vi "PatterningProgramV2.vi"() -> ()   [LabVIEW 2023]
uses:
  <vilib>/Platform/TimedLoop/XDataNode/timing_clust.ctl
  <vilib>/Platform/TimedLoop/XDataNode/nitl_modes.ctl
  <vilib>/Platform/TimedLoop/XDataNode/wakeup.ctl
  <vilib>/DAQmx/write.llb/DAQmx Write (Digital Bool 1Line 1Point).vi
  <vilib>/DAQmx/create/channels.llb/DAQmx Create Channel (DO-Digital Output).vi
  <vilib>/DAQmx/miscellaneous.llb/DAQmx Fill In Error Info.vi
  <vilib>/Platform/TimedLoop/XDataNode/XDataNode.xnode
  <vilib>/Platform/TimedLoop/XDataNode/XDNodeRunTimeDep.lvlib
  C:/Program Files (x86)/Control/SC3U.dll
  Program Files (x86)/Control/SC3U.dll
panel:
  out "Patterns Left":dbl
  out "Z Focus Positions":dbl[](array[numeric])
  out "Y Focus Positions":dbl[](array[numeric])
  out "X Focus Positions":dbl[](array[numeric])
  in  "Focus Position 4":bool
  in  "Focus Position 3":bool
  in  "Focus Position 2":bool
  in  "Focus Position 1":bool
  in  "stop":bool
  in  "450 nm":bool
  out "Boolean 3":bool
  in  "617 nm":bool
  out "Boolean 4":bool
  out "Patterning Time":dbl
  out "Pattern Spacing (mm)":dbl
  out "Well Spacing":dbl caption="Well Spacing (mm)"
  in  "START":bool
  in  "Pattern Time (s)":dbl=0.5 min=0.1 max=900.0
  in  "Well Columns":dbl=1.0 min=1.0 step=1.0
  in  "Well Rows":dbl=1.0 min=1.0 step=1.0
  in  "Pattern Columns":dbl=1.0 min=1.0 max=100.0 step=1.0
  in  "Pattern Rows":dbl=1.0 min=1.0 max=100.0 step=1.0
  in  "Select Objective Lens":u16(ring) items=["4X", "10X", "20X", "40X"]
  in  "Select Well Vessel":u16(ring) items=["Single Well", "6-Well Plate", "12-Well Plate", "24-Well Plate", "96-Well Plate"]
  in  "SC3U":refnum<k24>(container)
  out "ConnectStatus":bool
  out "ComUsing":i16
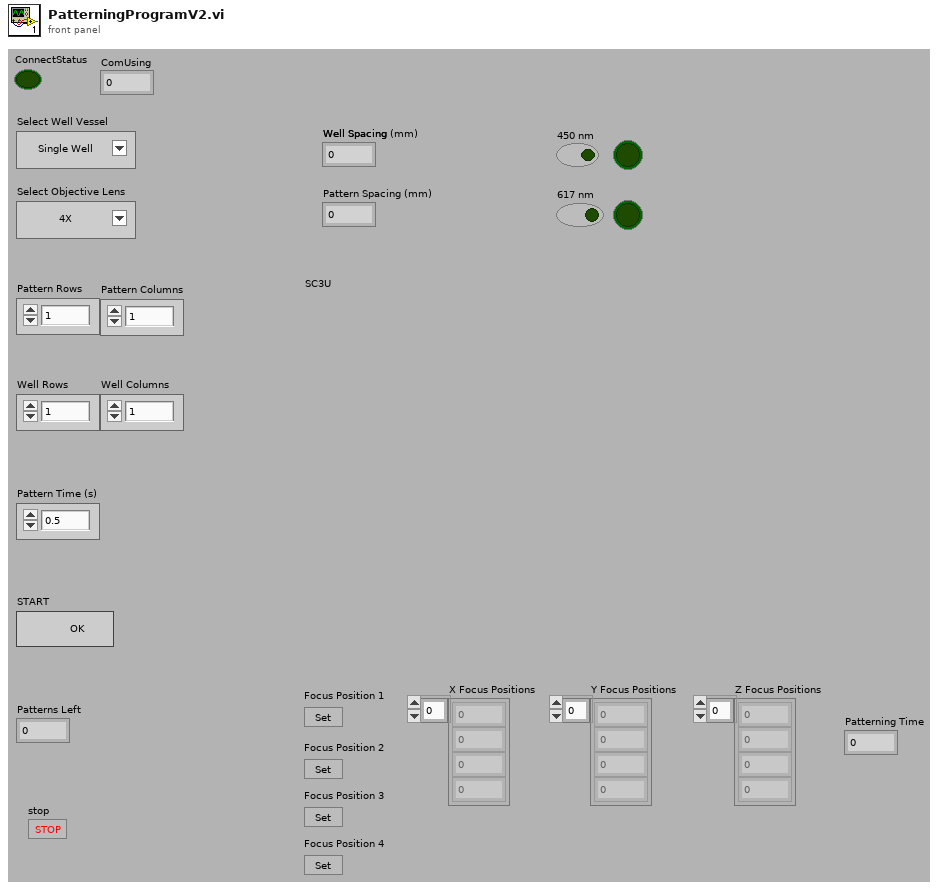
[diagram p1: front panel]
types:
  T1 = typedef "XDNodeRunTimeDep.lvlib/timing_clust.ctl" = cluster{"Expected End [f-1]":u64, "Actual End [f-1]":u64, "Finished Late? [f-1]":bool, "Expected End [i-1]":u64, "Actual End [i-1]":u64, "Finished Late? [i-1]":bool, "Expected Start [i]":u64, "Actual Start [i]":u64, "Expected Start [f]":u64, "Actual Start [f]":u64, "Source Name":string, "Structure Name":string, "Period":i64, "Deadline":i64, "Offset":i64, "Start":i64, "Priority":i32, "Timeout":i32, "Mode":T2, "Wakeup Reason":T3, "Error":errorcluster, "Source Type":string, "Secondary Source Type":string, "Global End Time":u64, "Global Start Time":u64, "Frame Duration":u64, "Iteration Duration":u64, "Assigned CPU":i32, "I/O Scan Engine Mode":u32}
  T2 = typedef "XDNodeRunTimeDep.lvlib/nitl_modes.ctl" = enum32{"No Change", "Process missed periods, maintain original phase", "Discard missed periods, maintain original phase", "Process missed periods, ignore original phase", "Discard missed periods, ignore original phase"}
  T3 = typedef "XDNodeRunTimeDep.lvlib/wakeup.ctl" = enum32{"Normal", "Aborted", "Asynchronous wakeup", "Timing source error", "Timed loop error", "Timeout"}
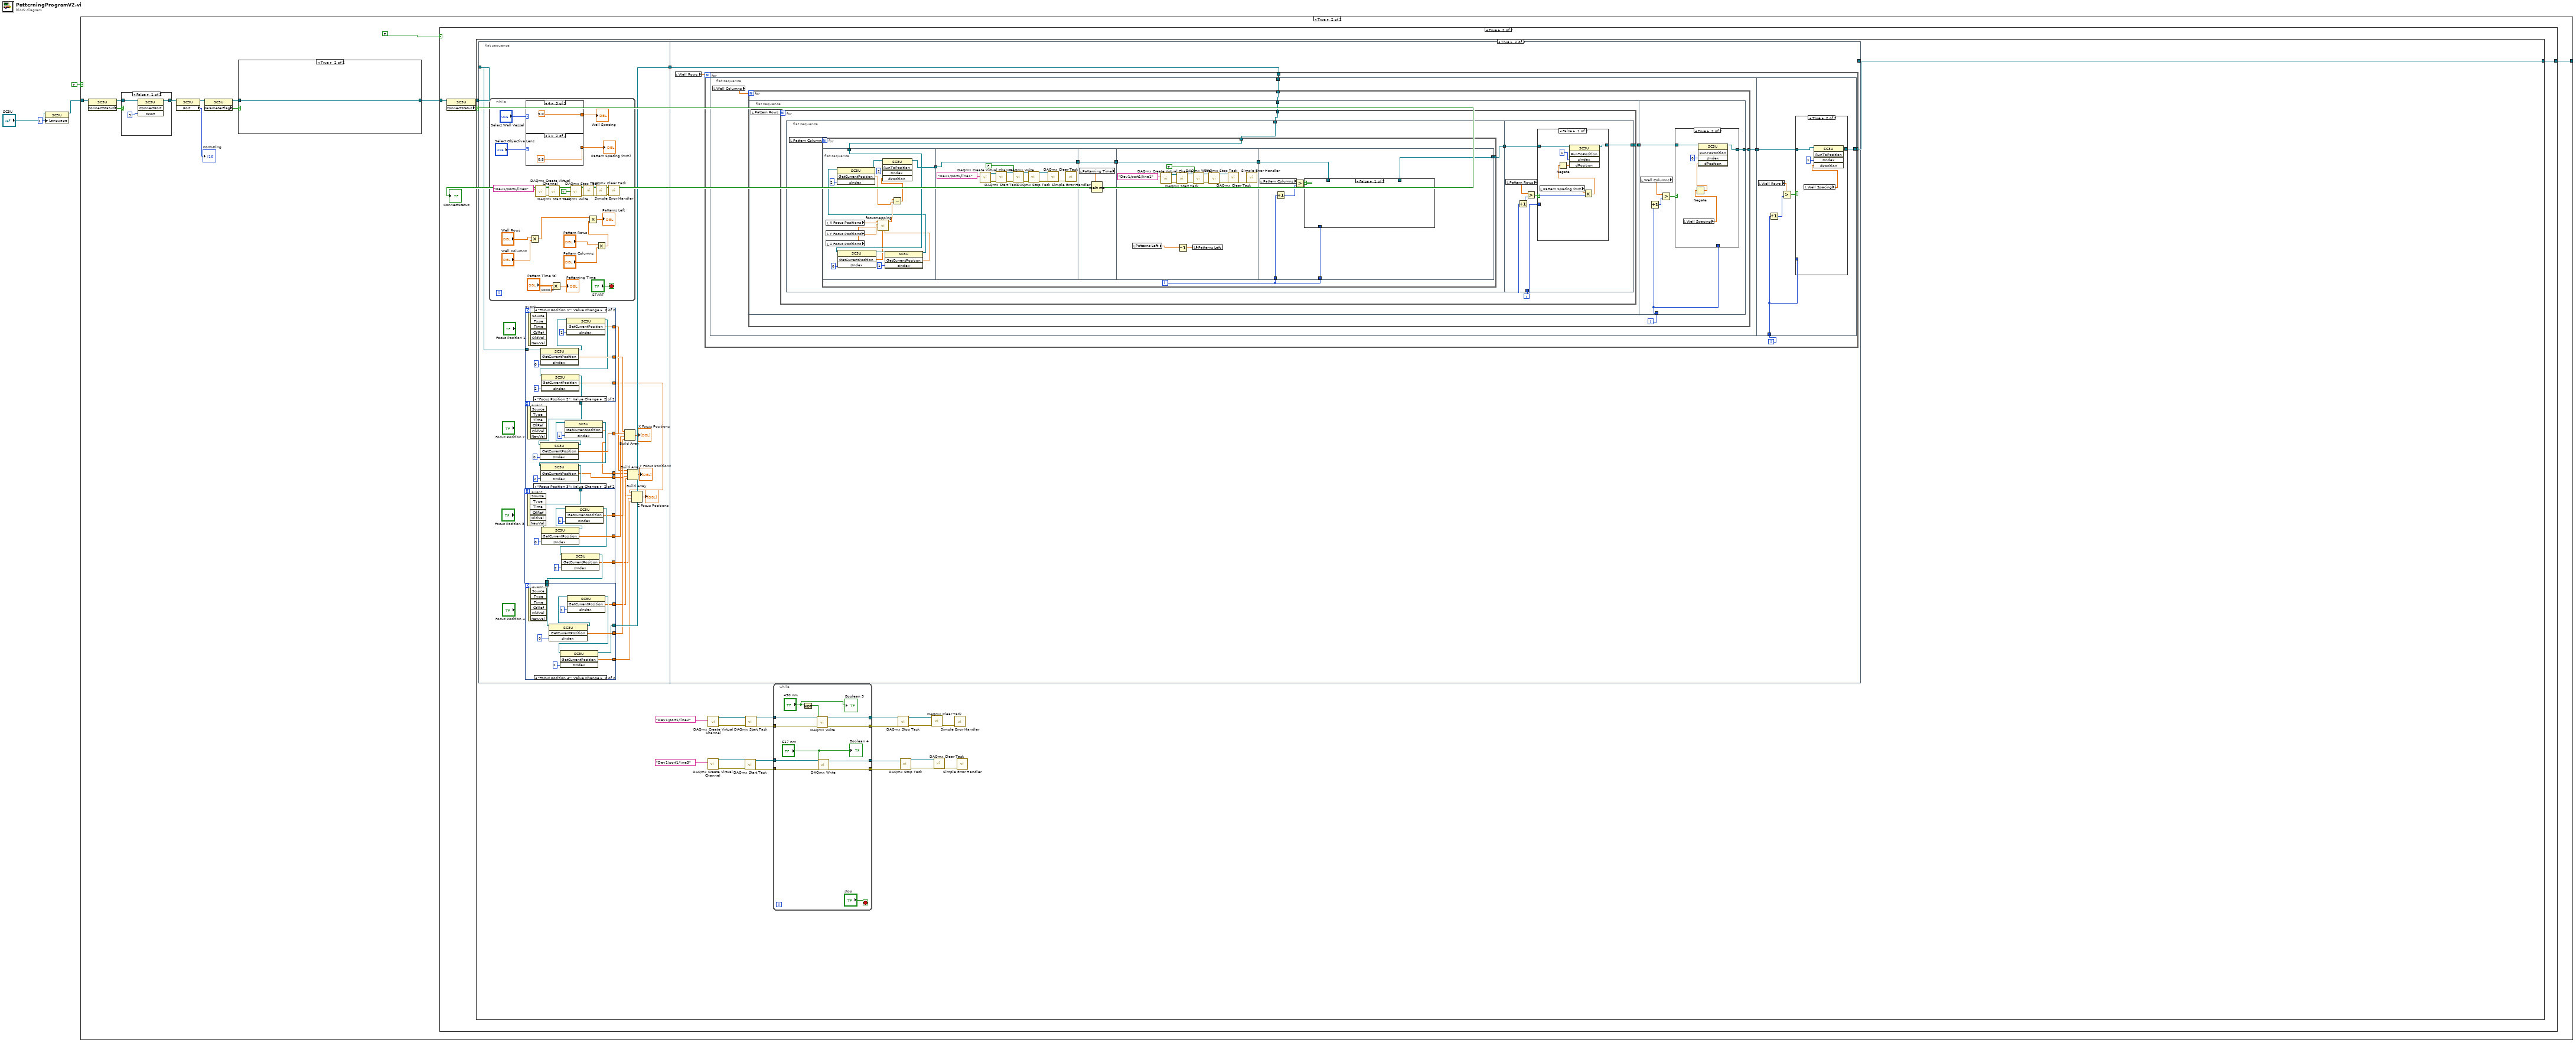
[diagram p0: block diagram]
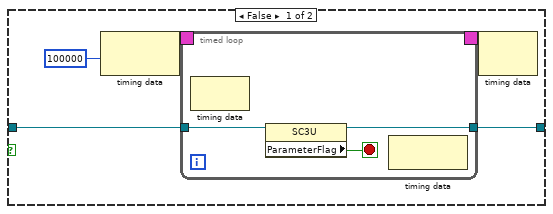
[diagram p3: hidden frame]
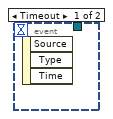
[diagram p7: hidden frame]
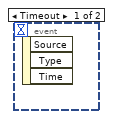
[diagram p8: hidden frame]
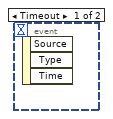
[diagram p9: hidden frame]
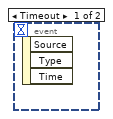
[diagram p10: hidden frame]
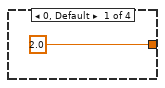
[diagram p11: hidden frame]
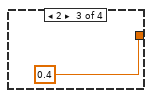
[diagram p12: hidden frame]
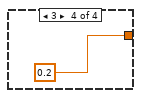
[diagram p13: hidden frame]
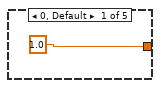
[diagram p14: hidden frame]
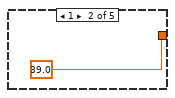
[diagram p15: hidden frame]
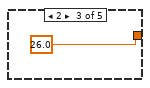
[diagram p16: hidden frame]
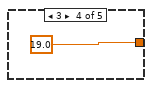
[diagram p17: hidden frame]
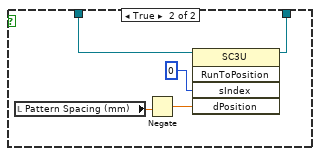
[diagram p18: hidden frame]
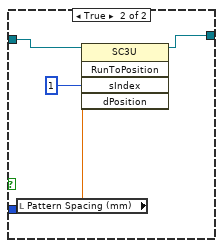
[diagram p19: hidden frame]
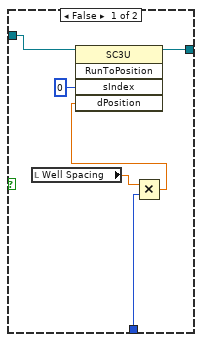
[diagram p20: hidden frame]
diagram:
  n1 = property class="SC3U"(reference="SC3U", "Language"=i16 1 ("intLanguage")) -> (reference out=w2:refnum<k24>)  [unwired: 1 in, 1 out]
  n2 = case shown="True" TRUE {
    tunnel: [_ w15] -> _
    tunnel: w2 -> [_ w13]
    frame False {
    }
    frame True {
      n3 = property class="SC3U"(reference=w13) -> (reference out=w12:refnum<k24>, "ConnectStatus"=w11:bool)  [unwired: 1 in, 1 out]
      n4 = case shown="False" w11 {
        tunnel: w12 -> [w33 w34]
        tunnel: [w32 w34] -> w10
        frame False {
          n5 = invoke class="SC3U" method="ConnectPort"(reference=w33, "sPort"=i16 5 ("ComUsing")) -> (reference out=w32:refnum<k24>)  [unwired: 2 in, 3 out]
        }
        frame True {
        }
      }
      n6 = property class="SC3U"(reference=w10) -> (reference out=w8:refnum<k24>, "Port"=→"ComUsing":i16)  [unwired: 1 in, 1 out]
      n7 = property class="SC3U"(reference=w8) -> (reference out=w7:refnum<k24>, "ParameterFlag"=w6:bool)  [unwired: 1 in, 1 out]
      n8 = case shown="True" w6 {
        tunnel: w7 -> [w17 w30]
        tunnel: [w16 w30] -> w14
        frame False {
          n9 = node-c288(i64 100000 ("周期")) -> (w20:T1)
          n10 = timed-loop {
            timing: w20 -> [_]
            timing-out: [_] -> w19
            tunnel: w17 -> [w23]
            tunnel: [w22] -> w16
            stop <- w21 stop-if-true
            n11 = node-c288() -> ()  [unwired: 1 in, 1 out]
            n12 = property class="SC3U"(reference=w23) -> (reference out=w22:refnum<k24>, "ParameterFlag"=w21:bool)  [unwired: 1 in, 1 out]
            n13 = node-c288() -> ()  [unwired: 1 in, 1 out]
          }
          n14 = node-c288(w19) -> ()  [unwired: 1 out]
        }
        frame True {
        }
      }
      n15 = case shown="True" TRUE {
        tunnel: w14 -> [_ w37]
        tunnel: [_ w38] -> w15
        frame False {
        }
        frame True {
          n16 = property class="SC3U"(reference=w37) -> (reference out=w36:refnum<k24>, "ConnectStatus"=w35:bool)  [unwired: 1 in, 1 out]
          "ConnectStatus" <- w35
          n17 = case shown="True" w35 {
            tunnel: w36 -> [_ w61]
            tunnel: [_ w59] -> w38
            frame False {
            }
            frame True {
              n18 = flat-sequence {
                tunnel: w61 -> [w93]
                tunnel: [w87] -> w60
                tunnel: w60 -> [w170]
                tunnel: [w169] -> w59
                frame #0 {
                  n19 = while {
                    stop <- "START" stop-if-true
                    n20 = case shown="1" "Select Objective Lens" {
                      tunnel: [2.0 ("Numeric") 0.8 ("Numeric") 0.4 ("Numeric") 0.2 ("Numeric")] -> w155
                      frame 0, Default {
                      }
                      frame 1 {
                      }
                      frame 2 {
                      }
                      frame 3 {
                      }
                    }
                    "Pattern Spacing (mm)" <- w155
                    n21 = case shown="4" "Select Well Vessel" {
                      tunnel: [1.0 ("Numeric") 39.0 ("Numeric") 26.0 ("Numeric") 19.0 ("Numeric") 9.0 ("Numeric")] -> w157
                      frame 0, Default {
                      }
                      frame 1 {
                      }
                      frame 2 {
                      }
                      frame 3 {
                      }
                      frame 4 {
                      }
                    }
                    "Well Spacing" <- w157
                    n22 = Multiply(x="Well Rows", y="Well Columns") -> (x*y=w136:dbl)
                    n23 = call-poly <vilib>:"DAQmx Create Virtual Channel.vi"("lines"=tag "Dev1/port1/line0") -> ("task out"=w151:refnum<k21>, "error out"=w149:errorcluster)  [unwired: 13 in]
                    n24 = call <vilib>:"DAQmx Start Task.vi"("task/channels in"=w151, "error in"=w149) -> ("task out"=w146:refnum<k21>, "error out"=w145:errorcluster)  [unwired: 12 in]
                    n25 = Multiply(x="Pattern Time (s)", y=1000.0) -> (x*y=→"Patterning Time":dbl)
                    n26 = call-poly <vilib>:"DAQmx Write.vi"("task/channels in"=w146, "data"=TRUE, "error in"=w145) -> ("task out"=w144:refnum<k21>, "error out"=w143:errorcluster)  [unwired: 10 in, 1 out]
                    n27 = call <vilib>:"DAQmx Stop Task.vi"("task/channels in"=w144, "error in"=w143) -> ("task out"=w150:refnum<k21>, "error out"=w148:errorcluster)  [unwired: 12 in]
                    n28 = call <vilib>:"DAQmx Clear Task.vi"("task in"=w150, "error in"=w148) -> ("error out"=w147:errorcluster)  [unwired: 13 in]
                    n29 = Multiply(x="Pattern Rows", y="Pattern Columns") -> (x*y=w135:dbl)
                    n30 = Multiply(x=w136, y=w135) -> (x*y=→"Patterns Left":dbl)
                    n31 = call <vilib>:"Simple Error Handler.vi"("error in (no error)"=w147) -> ()  [unwired: 4 in, 5 out]
                  }
                  n32 = event shown="[1] \"Focus Position 1\": Value Change" {
                    selector: _ -> [_ _]
                    dyn-events: _ -> [_ _]
                    timeout: _ -> [_ _]
                    tunnel: w93 -> [_ w132]
                    tunnel: [_ w131] -> w92
                    tunnel: [_ w126] -> w91
                    tunnel: [_ w125] -> w83
                    tunnel: [_ w124] -> w78
                    event Timeout {
                      n33 = event-data() -> ()  [unwired: 1 in, 3 out]
                    }
                    event "Focus Position 1": Value Change {
                      n34 = event-data() -> ()  [unwired: 1 in, 6 out]
                      n35 = invoke class="SC3U" method="GetCurrentPosition"(reference=w132, "sIndex"=i16 0) -> (reference out=w128:refnum<k24>, "GetCurrentPosition"=w131:dbl)  [unwired: 2 in, 2 out]
                      n36 = invoke class="SC3U" method="GetCurrentPosition"(reference=w128, "sIndex"=i16 1) -> (reference out=w127:refnum<k24>, "GetCurrentPosition"=w125:dbl)  [unwired: 2 in, 2 out]
                      n37 = invoke class="SC3U" method="GetCurrentPosition"(reference=w127, "sIndex"=i16 2) -> (reference out=w126:refnum<k24>, "GetCurrentPosition"=w124:dbl)  [unwired: 2 in, 2 out]
                    }
                  }
                  n38 = event shown="[1] \"Focus Position 2\": Value Change" {
                    selector: _ -> [_ _]
                    dyn-events: _ -> [_ _]
                    timeout: _ -> [_ _]
                    tunnel: w91 -> [_ w122]
                    tunnel: [_ w121] -> w90
                    tunnel: [_ w116] -> w89
                    tunnel: [_ w115] -> w82
                    tunnel: [_ w114] -> w77
                    event Timeout {
                      n39 = event-data() -> ()  [unwired: 1 in, 3 out]
                    }
                    event "Focus Position 2": Value Change {
                      n40 = event-data() -> ()  [unwired: 1 in, 6 out]
                      n41 = invoke class="SC3U" method="GetCurrentPosition"(reference=w122, "sIndex"=i16 0) -> (reference out=w118:refnum<k24>, "GetCurrentPosition"=w121:dbl)  [unwired: 2 in, 2 out]
                      n42 = invoke class="SC3U" method="GetCurrentPosition"(reference=w118, "sIndex"=i16 1) -> (reference out=w117:refnum<k24>, "GetCurrentPosition"=w115:dbl)  [unwired: 2 in, 2 out]
                      n43 = invoke class="SC3U" method="GetCurrentPosition"(reference=w117, "sIndex"=i16 2) -> (reference out=w116:refnum<k24>, "GetCurrentPosition"=w114:dbl)  [unwired: 2 in, 2 out]
                    }
                  }
                  n44 = event shown="[1] \"Focus Position 3\": Value Change" {
                    selector: _ -> [_ _]
                    dyn-events: _ -> [_ _]
                    timeout: _ -> [_ _]
                    tunnel: w89 -> [_ w112]
                    tunnel: [_ w106] -> w88
                    tunnel: [_ w111] -> w86
                    tunnel: [_ w105] -> w81
                    tunnel: [_ w104] -> w76
                    event Timeout {
                      n45 = event-data() -> ()  [unwired: 1 in, 3 out]
                    }
                    event "Focus Position 3": Value Change {
                      n46 = event-data() -> ()  [unwired: 1 in, 6 out]
                      n47 = invoke class="SC3U" method="GetCurrentPosition"(reference=w112, "sIndex"=i16 0) -> (reference out=w108:refnum<k24>, "GetCurrentPosition"=w111:dbl)  [unwired: 2 in, 2 out]
                      n48 = invoke class="SC3U" method="GetCurrentPosition"(reference=w108, "sIndex"=i16 1) -> (reference out=w107:refnum<k24>, "GetCurrentPosition"=w105:dbl)  [unwired: 2 in, 2 out]
                      n49 = invoke class="SC3U" method="GetCurrentPosition"(reference=w107, "sIndex"=i16 2) -> (reference out=w106:refnum<k24>, "GetCurrentPosition"=w104:dbl)  [unwired: 2 in, 2 out]
                    }
                  }
                  n50 = event shown="[1] \"Focus Position 4\": Value Change" {
                    selector: _ -> [_ _]
                    dyn-events: _ -> [_ _]
                    timeout: _ -> [_ _]
                    tunnel: w88 -> [_ w102]
                    tunnel: [_ w96] -> w87
                    tunnel: [_ w101] -> w85
                    tunnel: [_ w95] -> w80
                    tunnel: [_ w94] -> w75
                    event Timeout {
                      n51 = event-data() -> ()  [unwired: 1 in, 3 out]
                    }
                    event "Focus Position 4": Value Change {
                      n52 = event-data() -> ()  [unwired: 1 in, 6 out]
                      n53 = invoke class="SC3U" method="GetCurrentPosition"(reference=w102, "sIndex"=i16 0) -> (reference out=w98:refnum<k24>, "GetCurrentPosition"=w101:dbl)  [unwired: 2 in, 2 out]
                      n54 = invoke class="SC3U" method="GetCurrentPosition"(reference=w98, "sIndex"=i16 1) -> (reference out=w97:refnum<k24>, "GetCurrentPosition"=w95:dbl)  [unwired: 2 in, 2 out]
                      n55 = invoke class="SC3U" method="GetCurrentPosition"(reference=w97, "sIndex"=i16 2) -> (reference out=w96:refnum<k24>, "GetCurrentPosition"=w94:dbl)  [unwired: 2 in, 2 out]
                    }
                  }
                  n56 = Build Array(w92, w90, w86, w85) -> (→"X Focus Positions":dbl[])
                  n57 = Build Array(w83, w82, w81, w80) -> (→"Y Focus Positions":dbl[])
                  n58 = Build Array(w78, w77, w76, w75) -> (→"Z Focus Positions":dbl[])
                }
                frame #1 {
                  n59 = local read "Well Rows"() -> (w171:dbl)
                  n60 = for {
                    N: w171 -> [_]
                    tunnel: [w173] -> w169
                    tunnel: w170 -> [w172]
                    i -> [w175]
                    n61 = flat-sequence {
                      tunnel: [w177] -> w174
                      tunnel: w172 -> [w176]
                      tunnel: w175 -> [w299]
                      tunnel: w174 -> [w298]
                      tunnel: [w297] -> w173
                      frame #0 {
                        n62 = local read "Well Columns"() -> (w178:dbl)
                        n63 = for {
                          N: w178 -> [_]
                          tunnel: w176 -> [w182]
                          tunnel: [w179] -> w177
                          i -> [w181]
                          n64 = flat-sequence {
                            tunnel: w182 -> [w184]
                            tunnel: [w183] -> w180
                            tunnel: w181 -> [w281]
                            tunnel: w180 -> [w282]
                            tunnel: [w280] -> w179
                            frame #0 {
                              n65 = local read "Pattern Rows"() -> (w185:dbl)
                              n66 = for {
                                N: w185 -> [_]
                                tunnel: w184 -> [w189]
                                tunnel: [w186] -> w183
                                i -> [w188]
                                n67 = flat-sequence {
                                tunnel: w189 -> [w191]
                                tunnel: [w190] -> w187
                                tunnel: w188 -> [w265]
                                tunnel: w187 -> [w264]
                                tunnel: [w263] -> w186
                                frame #0 {
                                n68 = local read "Pattern Columns"() -> (w192:dbl)
                                n69 = for {
                                N: w192 -> [_]
                                tunnel: w191 -> [w197]
                                tunnel: [w199] -> w190
                                i -> [w198]
                                n70 = flat-sequence {
                                tunnel: w197 -> [w204]
                                tunnel: [w215] -> w193
                                tunnel: [w217] -> w194
                                tunnel: w193 -> [w217]
                                tunnel: [w229] -> w195
                                tunnel: w194 -> [w229]
                                tunnel: [w233] -> w196
                                tunnel: w195 -> [w233]
                                tunnel: w198 -> [w247]
                                tunnel: [w249] -> w199
                                tunnel: w198 -> [w248]
                                tunnel: w196 -> [w245]
                                frame #0 {
                                n71 = local read "X Focus Positions"() -> (w210:dbl[])
                                n72 = local read "Y Focus Positions"() -> (w209:dbl[])
                                n73 = local read "Z Focus Positions"() -> (w208:dbl[])
                                n74 = invoke class="SC3U" method="GetCurrentPosition"(reference=w204, "sIndex"=i16 0) -> (reference out=w203:refnum<k24>, "GetCurrentPosition"=w201:dbl)  [unwired: 2 in, 2 out]
                                n75 = invoke class="SC3U" method="GetCurrentPosition"(reference=w203, "sIndex"=i16 1) -> (reference out=w202:refnum<k24>, "GetCurrentPosition"=w200:dbl)  [unwired: 2 in, 2 out]
                                n76 = invoke class="SC3U" method="GetCurrentPosition"(reference=w202, "sIndex"=i16 2) -> (reference out=w213:refnum<k24>, "GetCurrentPosition"=w212:dbl)  [unwired: 2 in, 2 out]
                                n77 = call "focusmapping.vi"("Current Y Position"=w200, "Current X Position"=w201, "Z Locations"=w208, "Y Locations"=w209, "X Locations"=w210) -> ("MoveTo Z"=w207:dbl)  [unwired: 6 in]
                                n78 = Subtract(x=w207, y=w212) -> (x-y=w211:dbl)
                                n79 = invoke class="SC3U" method="RunToPosition"(reference=w213, "sIndex"=i16 2, "dPosition"=w211) -> (reference out=w215:refnum<k24>)  [unwired: 2 in, 4 out]
                                }
                                frame #1 {
                                n80 = call-poly <vilib>:"DAQmx Create Virtual Channel.vi"("lines"=tag "Dev1/port1/line1") -> ("task out"=w227:refnum<k21>, "error out"=w228:errorcluster)  [unwired: 13 in]
                                n81 = call <vilib>:"DAQmx Start Task.vi"("task/channels in"=w227, "error in"=w228) -> ("task out"=w222:refnum<k21>, "error out"=w224:errorcluster)  [unwired: 12 in]
                                n82 = call-poly <vilib>:"DAQmx Write.vi"("task/channels in"=w222, "data"=FALSE, "error in"=w224) -> ("task out"=w221:refnum<k21>, "error out"=w223:errorcluster)  [unwired: 10 in, 1 out]
                                n83 = call <vilib>:"DAQmx Stop Task.vi"("task/channels in"=w221, "error in"=w223) -> ("task out"=w220:refnum<k21>, "error out"=w225:errorcluster)  [unwired: 12 in]
                                n84 = call <vilib>:"DAQmx Clear Task.vi"("task in"=w220, "error in"=w225) -> ("error out"=w226:errorcluster)  [unwired: 13 in]
                                n85 = call <vilib>:"Simple Error Handler.vi"("error in (no error)"=w226) -> ()  [unwired: 4 in, 5 out]
                                }
                                frame #2 {
                                n86 = local read "Patterning Time"() -> (w230:dbl)
                                n87 = Wait (ms)(milliseconds to wait=w230) -> ()  [unwired: 1 out]
                                }
                                frame #3 {
                                n88 = local read "Patterns Left"() -> (w231:dbl)
                                n89 = call-poly <vilib>:"DAQmx Create Virtual Channel.vi"("lines"=tag "Dev1/port1/line1") -> ("task out"=w237:refnum<k21>, "error out"=w236:errorcluster)  [unwired: 13 in]
                                n90 = call <vilib>:"DAQmx Start Task.vi"("task/channels in"=w237, "error in"=w236) -> ("task out"=w242:refnum<k21>, "error out"=w240:errorcluster)  [unwired: 12 in]
                                n91 = Decrement(x=w231) -> (x-1=w232:dbl)
                                n92 = local write "Patterns Left"(w232) -> ()
                                n93 = call-poly <vilib>:"DAQmx Write.vi"("task/channels in"=w242, "data"=TRUE, "error in"=w240) -> ("task out"=w243:refnum<k21>, "error out"=w241:errorcluster)  [unwired: 10 in, 1 out]
                                n94 = call <vilib>:"DAQmx Stop Task.vi"("task/channels in"=w243, "error in"=w241) -> ("task out"=w244:refnum<k21>, "error out"=w239:errorcluster)  [unwired: 12 in]
                                n95 = call <vilib>:"DAQmx Clear Task.vi"("task in"=w244, "error in"=w239) -> ("error out"=w238:errorcluster)  [unwired: 13 in]
                                n96 = call <vilib>:"Simple Error Handler.vi"("error in (no error)"=w238) -> ()  [unwired: 4 in, 5 out]
                                }
                                frame #4 {
                                n97 = local read "Pattern Columns"() -> (w251:dbl)
                                n98 = Increment(x=w247) -> (x+1=w246:i32)
                                n99 = Greater?(x=w251, y=w246) -> (0:w250:bool)
                                n100 = case shown="False" w250 {
                                tunnel: w245 -> [w256 w262]
                                tunnel: [w252 w260] -> w249
                                tunnel: w248 -> [w254 _]
                                frame False {
                                n101 = local read "Pattern Spacing (mm)"() -> (w255:dbl)
                                n102 = Multiply(x=w255, y=w254) -> (x*y=w253:dbl)
                                n103 = invoke class="SC3U" method="RunToPosition"(reference=w256, "sIndex"=i16 0, "dPosition"=w253) -> (reference out=w252:refnum<k24>)  [unwired: 2 in, 4 out]
                                }
                                frame True {
                                n104 = local read "Pattern Spacing (mm)"() -> (w259:dbl)
                                n105 = Negate(x=w259) -> (-x=w258:dbl)
                                n106 = invoke class="SC3U" method="RunToPosition"(reference=w262, "sIndex"=i16 0, "dPosition"=w258) -> (reference out=w260:refnum<k24>)  [unwired: 2 in, 4 out]
                                }
                                }
                                }
                                }
                                }
                                }
                                frame #1 {
                                n107 = local read "Pattern Rows"() -> (w268:dbl)
                                n108 = Increment(x=w265) -> (x+1=w266:i32)
                                n109 = Greater?(x=w268, y=w266) -> (0:w267:bool)
                                n110 = case shown="False" w267 {
                                tunnel: w265 -> [w273 _]
                                tunnel: w264 -> [w272 w277]
                                tunnel: [w269 w276] -> w263
                                frame False {
                                n111 = local read "Pattern Spacing (mm)"() -> (w275:dbl)
                                n112 = Multiply(x=w275, y=w273) -> (x*y=w270:dbl)
                                n113 = Negate(x=w270) -> (-x=w271:dbl)
                                n114 = invoke class="SC3U" method="RunToPosition"(reference=w272, "sIndex"=i16 1, "dPosition"=w271) -> (reference out=w269:refnum<k24>)  [unwired: 2 in, 4 out]
                                }
                                frame True {
                                n115 = local read "Pattern Spacing (mm)"() -> (w278:dbl)
                                n116 = invoke class="SC3U" method="RunToPosition"(reference=w277, "sIndex"=i16 1, "dPosition"=w278) -> (reference out=w276:refnum<k24>)  [unwired: 2 in, 4 out]
                                }
                                }
                                }
                                }
                              }
                            }
                            frame #1 {
                              n117 = local read "Well Columns"() -> (w283:dbl)
                              n118 = Increment(x=w281) -> (x+1=w284:i32)
                              n119 = Greater?(x=w283, y=w284) -> (0:w285:bool)
                              n120 = case shown="True" w285 {
                                tunnel: w282 -> [w287 w293]
                                tunnel: w281 -> [w289 _]
                                tunnel: [w286 w292] -> w280
                                frame False {
                                n121 = local read "Well Spacing"() -> (w290:dbl)
                                n122 = Multiply(x=w290, y=w289) -> (x*y=w288:dbl)
                                n123 = invoke class="SC3U" method="RunToPosition"(reference=w287, "sIndex"=i16 0, "dPosition"=w288) -> (reference out=w286:refnum<k24>)  [unwired: 2 in, 4 out]
                                }
                                frame True {
                                n124 = local read "Well Spacing"() -> (w295:dbl)
                                n125 = Negate(x=w295) -> (-x=w294:dbl)
                                n126 = invoke class="SC3U" method="RunToPosition"(reference=w293, "sIndex"=i16 0, "dPosition"=w294) -> (reference out=w292:refnum<k24>)  [unwired: 2 in, 4 out]
                                }
                              }
                            }
                          }
                        }
                      }
                      frame #1 {
                        n127 = local read "Well Rows"() -> (w301:dbl)
                        n128 = Increment(x=w299) -> (x+1=w300:i32)
                        n129 = Greater?(x=w301, y=w300) -> (0:w302:bool)
                        n130 = case shown="True" w302 {
                          tunnel: w299 -> [w305 _]
                          tunnel: w298 -> [w304 w311]
                          tunnel: [w303 w310] -> w297
                          frame False {
                            n131 = local read "Well Spacing"() -> (w308:dbl)
                            n132 = Multiply(x=w308, y=w305) -> (x*y=w306:dbl)
                            n133 = Negate(x=w306) -> (-x=w307:dbl)
                            n134 = invoke class="SC3U" method="RunToPosition"(reference=w304, "sIndex"=i16 1, "dPosition"=w307) -> (reference out=w303:refnum<k24>)  [unwired: 2 in, 4 out]
                          }
                          frame True {
                            n135 = local read "Well Spacing"() -> (w312:dbl)
                            n136 = invoke class="SC3U" method="RunToPosition"(reference=w311, "sIndex"=i16 1, "dPosition"=w312) -> (reference out=w310:refnum<k24>)  [unwired: 2 in, 4 out]
                          }
                        }
                      }
                    }
                  }
                }
              }
              n137 = call-poly <vilib>:"DAQmx Create Virtual Channel.vi"("lines"=tag "Dev1/port1/line3") -> ("task out"=w55:refnum<k21>, "error out"=w54:errorcluster)  [unwired: 13 in]
              n138 = call-poly <vilib>:"DAQmx Create Virtual Channel.vi"("lines"=tag "Dev1/port1/line2") -> ("task out"=w58:refnum<k21>, "error out"=w57:errorcluster)  [unwired: 13 in]
              n139 = call <vilib>:"DAQmx Start Task.vi"("task/channels in"=w55, "error in"=w54) -> ("task out"=w42:refnum<k21>, "error out"=w41:errorcluster)  [unwired: 12 in]
              n140 = call <vilib>:"DAQmx Start Task.vi"("task/channels in"=w58, "error in"=w57) -> ("task out"=w46:refnum<k21>, "error out"=w45:errorcluster)  [unwired: 12 in]
              n141 = while {
                tunnel: w46 -> [w71]
                tunnel: w45 -> [w70]
                tunnel: [w69] -> w44
                tunnel: [w68] -> w43
                tunnel: w42 -> [w67]
                tunnel: w41 -> [w66]
                tunnel: [w65] -> w40
                tunnel: [w64] -> w39
                stop <- "stop" stop-if-true
                n142 = Not(x="450 nm") -> (.not. x?=w63:bool)
                n143 = call-poly <vilib>:"DAQmx Write.vi"("task/channels in"=w71, "data"=w63, "error in"=w70) -> ("task out"=w69:refnum<k21>, "error out"=w68:errorcluster)  [unwired: 10 in, 1 out]
                n144 = call-poly <vilib>:"DAQmx Write.vi"("task/channels in"=w67, "data"="617 nm", "error in"=w66) -> ("task out"=w65:refnum<k21>, "error out"=w64:errorcluster)  [unwired: 10 in, 1 out]
                "Boolean 3" <- "450 nm"
                "Boolean 4" <- "617 nm"
              }
              n145 = call <vilib>:"DAQmx Stop Task.vi"("task/channels in"=w44, "error in"=w43) -> ("task out"=w52:refnum<k21>, "error out"=w51:errorcluster)  [unwired: 12 in]
              n146 = call <vilib>:"DAQmx Stop Task.vi"("task/channels in"=w40, "error in"=w39) -> ("task out"=w49:refnum<k21>, "error out"=w48:errorcluster)  [unwired: 12 in]
              n147 = call <vilib>:"DAQmx Clear Task.vi"("task in"=w52, "error in"=w51) -> ("error out"=w50:errorcluster)  [unwired: 13 in]
              n148 = call <vilib>:"DAQmx Clear Task.vi"("task in"=w49, "error in"=w48) -> ("error out"=w47:errorcluster)  [unwired: 13 in]
              n149 = call <vilib>:"Simple Error Handler.vi"("error in (no error)"=w50) -> ()  [unwired: 4 in, 5 out]
              n150 = call <vilib>:"Simple Error Handler.vi"("error in (no error)"=w47) -> ()  [unwired: 4 in, 5 out]
            }
          }
        }
      }
    }
  }
